vi "HTTPErrCheck.vi"(8 "error in (no error)":errorcluster, 11 "Comm":T1) -> (0 "error out":errorcluster, 3 "error":i32)   [LabVIEW 2016]
uses:
  HTTPComm.ctl
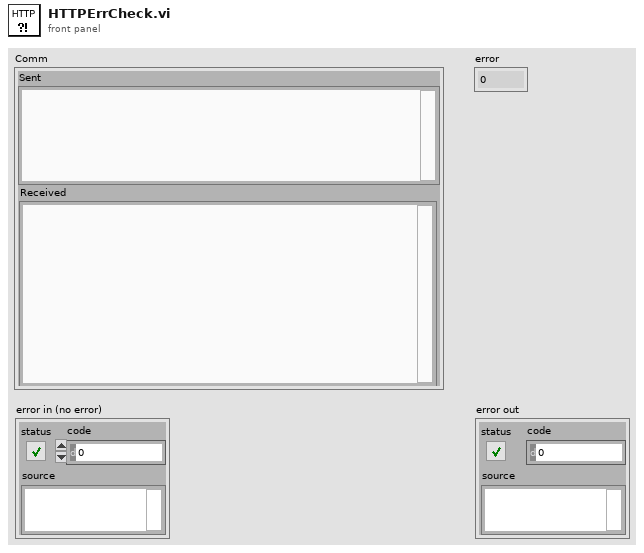
[diagram p1: front panel]
types:
  T1 = typedef "HTTPComm.ctl" = cluster{"url":string, "sent headers":string, "sent body":string, "headers":string, "body":string, "Sent":string, "Received":string}
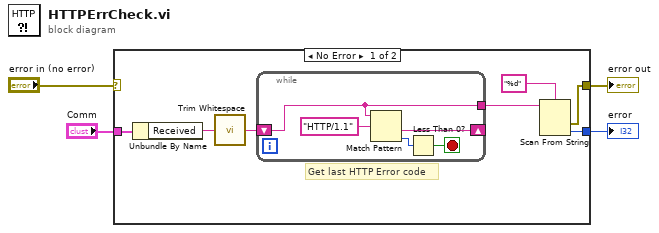
[diagram p0: block diagram]
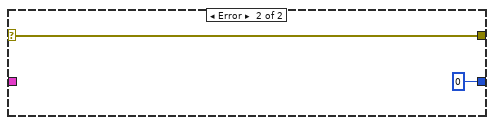
[diagram p2: hidden frame]
diagram:
  n1 = case shown="No Error" "error in (no error)" {
    selector: "error in (no error)" -> [_ w18]
    tunnel: "Comm" -> [w8 _]
    tunnel: [w5 w18] -> w3
    tunnel: [w6 0] -> w1
    frame No Error {
      # "Get last HTTP Error code"
      n2 = Unbundle By Name(w8) -> ("Received"=w9:string)
      n3 = call <vilib>:"Trim Whitespace.vi"("string"=w9) -> ("trimmed string"=w10:string)  [unwired: 1 in]
      n4 = while {
        shift-right: [w13] -> _
        shift-left: w10 -> [w12]
        tunnel: [w12] -> w11
        stop <- w15 stop-if-true
        n5 = Match Pattern(string=w12, regular expression="HTTP/1.1") -> (after substring=w13:string, offset past match=w14:i32)  [unwired: 1 in, 2 out]
        n6 = Less Than 0?(x=w14) -> (x < 0?=w15:bool)
      }
      n7 = Scan From String(format string="%d", input string=w11) -> (error out=w5:errorcluster, output 1=w6:i32)  [unwired: 3 in, 2 out]
    }
    frame Error {
    }
  }
  "error out" <- w3
  "error" <- w1
